vi "ComputePiezoParameters.vi"(0 "Frame per fringe":dbl=5.0 format="%.2f", 1 "Wavelength":dbl[unit]=2.2e-06 format="%.2f", 2 "READOUT":T2, 4 "Autcollimation":bool) -> (5 "OPD stroke":dbl[unit], 6 "WAVE":T1={"Speed"=0.0, "Stiffness (0.95)"=0.95, "Linear Stroke"=0.0, "Delay"=0.0} {"Delay" format="%.2f"; "Linear Stroke" format="%.2f"; "Stiffness (0.95)" format="%.2f"; "Speed" format="%.2f"})   [LabVIEW 2009]
uses:
  Instruments/Nicmos/Controls/NICMOS.READOUT.ctl
  Instruments/Piezo/Controls/PIEZO.WAVE.ctl
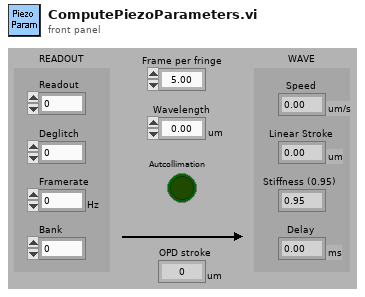
[diagram p1: front panel]
types:
  T1 = typedef "PIEZO.WAVE.ctl" = cluster{"Speed":dbl[unit], "Stiffness (0.95)":dbl, "Linear Stroke":dbl[unit], "Delay":dbl[unit]}
  T2 = typedef "NICMOS.READOUT.ctl" = cluster{"Readout":i32, "Deglitch":i32, "Framerate":dbl[unit], "Bank":i32}
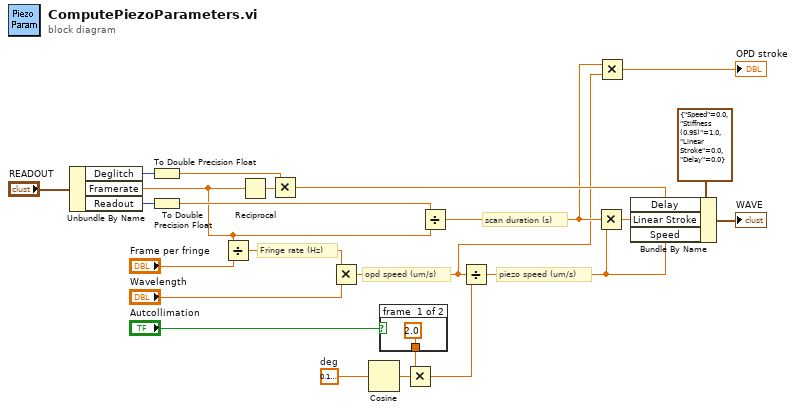
[diagram p0: block diagram]
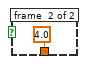
[diagram p2: hidden frame]
diagram:
  w23 = dbl[unit] 0.17453292519943295  # deg
  # "Fringe rate (Hz)"
  # "scan duration (s)"
  # "piezo speed (um/s)"
  # "opd speed (um/s)"
  n1 = Unbundle By Name("READOUT") -> ("Deglitch"=w11:i32, "Framerate"=w10:dbl[unit], "Readout"=w9:i32)
  n2 = To Double Precision Float(number=w11) -> (double precision float=w16:dbl)
  n3 = To Double Precision Float(number=w9) -> (double precision float=w18:dbl)
  n4 = Divide(x=w10, y="Frame per fringe") -> (x/y=w17:dbl[unit])
  n5 = Reciprocal(x=w10) -> (1/x=w15:dbl[unit])
  n6 = Multiply(x=w16, y=w15) -> (x*y=w5:dbl[unit])
  n7 = Multiply(x=w17, y="Wavelength") -> (x*y=w2:dbl[unit])
  n8 = Cosine(x=w23) -> (cos(x)=w21:dbl)
  n9 = case shown="False" "Autcollimation" {
    tunnel: [2.0 ("x") 4.0 ("x")] -> w20
    frame #0 {
    }
    frame #1 {
    }
  }
  n10 = Multiply(x=w21, y=w20) -> (x*y=w22:dbl)
  n11 = Divide(x=w18, y=w10) -> (x/y=w3:dbl[unit])
  n12 = Divide(x=w2, y=w22) -> (x/y=w4:dbl[unit])
  n13 = Multiply(x=w3, y=w4) -> (x*y=w6:dbl[unit])
  n14 = Multiply(x=w3, y=w2) -> (x*y=→"OPD stroke":dbl[unit])
  n15 = Bundle By Name(cluster=T1 {"Speed"=0.0, "Stiffness (0.95)"=1.0, "Linear Stroke"=0.0, "Delay"=0.0} ("WAVE"), "Delay"=w5, "Linear Stroke"=w6, "Speed"=w4) -> (→"WAVE":T1)
